vi "MatlabEventStructToLabviewData.vi"(0 "Event Variant":variant, 5 "Value to update (or object type)":variant) -> (4 "Value":variant, 6 "Name":string, 10 "Category":string)   [LabVIEW 2017]
uses:
  Types/MatlabEventStruct.ctl
  Types/MatlabDataBundle.ctl
  Types/MatlabDataType.ctl
  Types/MatlabDataContainerType.ctl
panel:
  out "DataIndex":dbl
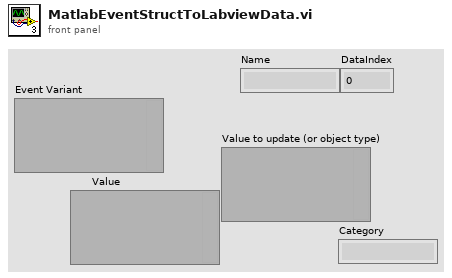
[diagram p1: front panel]
types:
  T1 = typedef "MatlabEventStruct.ctl" = cluster{"Name":string, "DataIndex":dbl, "Category":string, "Matlab Param Data":T2[]}
  T2 = typedef "MatlabDataBundle.ctl" = cluster{"MatlabType":T3, "Value":variant, "Name":string, "Typename":string, "Container Type":T4}
  T3 = typedef "MatlabDataType.ctl" = enum16{"NotAMatlabType", "Real", "Complex", "String", "Boolean"}
  T4 = typedef "MatlabDataContainerType.ctl" = enum16{"Numeric Value", "Numeric Array", "Waveform"}
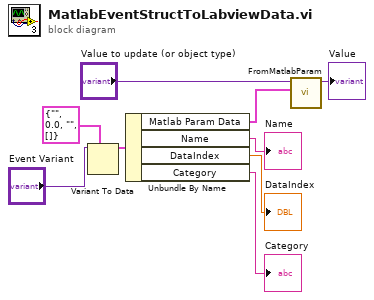
[diagram p0: block diagram]
diagram:
  n1 = Variant To Data(type=T1 {"Name"="", "DataIndex"=0.0, "Category"="", "Matlab Param Data"=[]} ("MatlabEvent"), Variant="Event Variant") -> (data=w7:T1)  [unwired: 1 in, 1 out]
  n2 = Unbundle By Name(w7) -> ("Matlab Param Data"=w8:T2[], "Name"=→"Name":string, "DataIndex"=→"DataIndex":dbl, "Category"=→"Category":string)
  n3 = call "FromMatlabParam.vi"("Matlab Param Data"=w8, "Type (or value to update)"="Value to update (or object type)") -> ("Value"=→"Value":variant)  [unwired: 9 in]
